vi "BoolToU8.vi"(11 "Boolean":bool=TRUE) -> (3 "Numeric":u8)   [LabVIEW 2012]
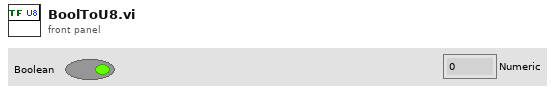
[diagram p1: front panel]
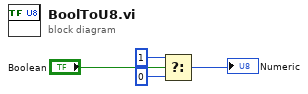
[diagram p0: block diagram]
diagram:
  n1 = Select(t=u8 1, s="Boolean", f=u8 0) -> (s? t:f=→"Numeric":u8)
